vi "ExCenterStripSpecFwIN.vi"() -> ()   [LabVIEW 2010]
panel:
  in  "Filter":i16=1 min=1 max=100 step=1
  in  "Wavelength":dbl=546.0 format="%.2f"
  in  "Grating Speed":dbl=2000.0 min=1.0 step=1.0 format="%.2f"
  in  "Grating number":i16=1 min=1 max=100 step=1
  out "Strip":sgl[](graph)
  in  "Temperature":dbl=-10.0 format="%.2f"
  in  "Exposure":dbl=0.5 min=0.0 step=0.001 format="%.3f"
  in  "stop":bool
  out "error out":errorcluster
  in  "error in (no error)":errorcluster
  # "ExCenterStripSpecFwIN.vi (InSpectrum)\nCamera, Spectrometer and Filter Wheel control of the InSpectrum.  This vi will open the camera, spectrograph and filter wheel.  It will then move the grating to the Wavelength and set the filter.  Data will then be collected and displayed until the STOP button is hit."
  # "NOTES:\nA properly configured spectometer .ini must be present in the LabVIEW folder for spectrograph operation.\n\nConsult the Toolkit documentation for more information on how to configure this file."
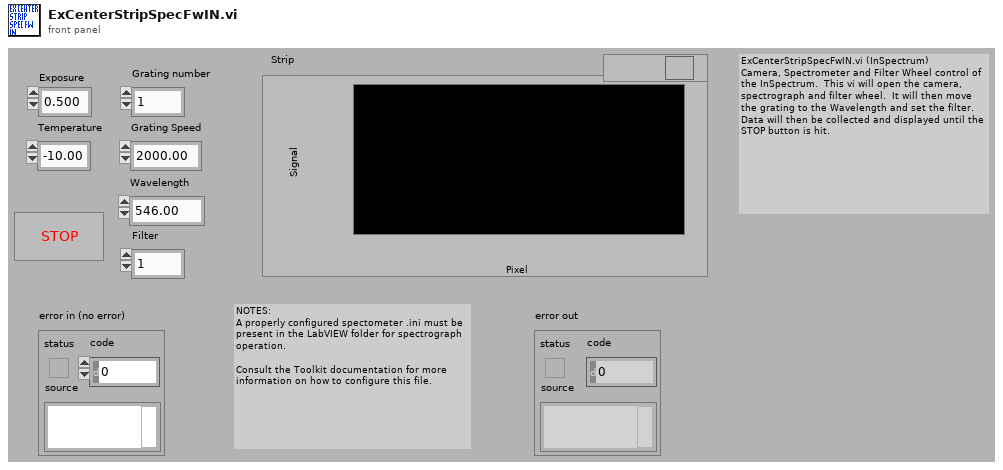
[diagram p1: front panel]
types:
  T1 = cluster{"acquire focus mode":u32, "Exposure":dbl, "Number of Images":u32, "Software accumulation":u32}
  T2 = cluster{"Camera Handle":u32, "Pulser Handle":u32, "File Handle":u32, "Display Handle":u32, "Image Handle":u32}
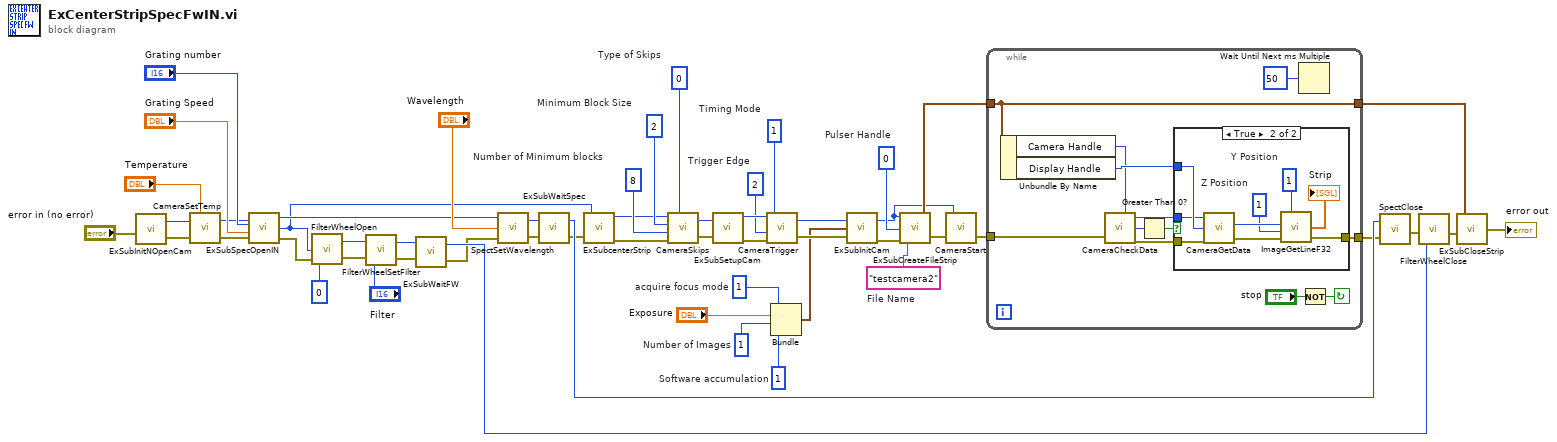
[diagram p0: block diagram]
diagram:
  w26 = u32 0  # Pulser Handle
  w31 = u32 1  # acquire focus mode
  w30 = u32 1  # Number of Images
  w29 = u32 1  # Software accumulation
  w28 = u32 1  # Timing Mode
  w32 = u32 2  # Trigger Edge
  w34 = u32 0  # Type of Skips
  w35 = u32 2  # Minimum Block Size
  w33 = u32 8  # Number of Minimum blocks
  w24 = "testcamera2"  # File Name
  n1 = call "ExSubInitNOpenCam.vi"("error in (no error)"="error in (no error)") -> ("Camera Handle"=w12:u32, "error out"=w13:errorcluster)
  n2 = call <userlib>:"CameraSetTemp.vi"("error in (no error)"=w13, "Temperature"="Temperature", "Camera Handle"=w12) -> ("error out"=w9:errorcluster, "Camera Handle"=w10:u32)
  n3 = call "ExSubSpecOpenIN.vi"("error in (no error)"=w9, "Grating speed"="Grating Speed", "Grating number"="Grating number", "Camera Handles"=w10) -> ("error out"=w18:errorcluster, "Camera Handle"=w16:u32, "Spectrometer Handle"=w38:u32)
  n4 = call <userlib>:"FilterWheelOpen.vi"("error in"=w18, "Device Handle"=w16, "Filter Wheel ID"=0) -> ("error out"=w17:errorcluster, "Filter Wheel Handlle"=w14:u32)
  n5 = call <userlib>:"FilterWheelSetFilter.vi"("error in"=w17, "Filter"="Filter", "Filter Wheel Handle"=w14) -> ("error out"=w7:errorcluster, "Filter Wheel Handle"=w5:u32)  [unwired: 1 in]
  n6 = call "ExSubWaitFW.vi"("error in (no error)"=w7, "Filter Wheel Handle"=w5) -> ("error out"=w6:errorcluster, "Filter Wheel handle"=w8:u32)
  n7 = call <userlib>:"SpectSetWavelength.vi"("error in"=w6, "Wavelength"="Wavelength", "Spectrometer Handle"=w38) -> ("error out"=w40:errorcluster, "Spectrumeter Handle"=w39:u32)
  n8 = call "ExSubWaitSpec.vi"("error in (no error)"=w40, "Spectrometer Handle"=w39) -> ("error out"=w23:errorcluster, "Spectrometer handle"=w37:u32)
  n9 = call "ExSubcenterStrip.vi"("error in (no error)"=w23, "Camera Handle"=w16) -> ("error out"=w21:errorcluster, "Camera Handle"=w22:u32)
  n10 = call <userlib>:"CameraSkips.vi"("Camera Handle"=w22, "Minimum Block Size"=w35, "Number of Minimum blocks"=w33, "error in"=w21, "Type of Skips"=w34) -> ("Camera Handle"=w46:u32, "error out"=w45:errorcluster)
  n11 = call "ExSubSetupCam.vi"("error in (no error)"=w45, "Camera Handle"=w46) -> ("error out"=w19:errorcluster, "Camera Handle"=w49:u32)
  n12 = call <userlib>:"CameraTrigger.vi"("error in"=w19, "Trigger Edge"=w32, "Timing Mode"=w28, "Camera Handle"=w49) -> ("error out"=w50:errorcluster, "Camera Handle"=w48:u32)
  n13 = Bundle("acquire focus mode"=w31, "Exposure"="Exposure", "Number of Images"=w30, "Software accumulation"=w29) -> (w27:T1)  [unwired: 1 in]
  n14 = call "ExSubInitCam.vi"("error in (no error)"=w50, "Camera Information"=w27, "Camera Handle"=w48) -> ("error out"=w20:errorcluster, "Camera Handle"=w25:u32)
  n15 = call "ExSubCreateFileStrip.vi"("error in (no error)"=w20, "File and Display Name"=w24, "Pulser Handle"=w26, "Camera Handle"=w25) -> ("error out"=w44:errorcluster, "Handles Out"=w52:T2)
  n16 = call <userlib>:"CameraStart.vi"("error in"=w44, "Camera Handle"=w25) -> ("error out"=w47:errorcluster)  [unwired: 1 out]
  n17 = while {
    tunnel: w52 -> [w63]
    tunnel: w47 -> [w62]
    tunnel: [w60] -> w36
    tunnel: [w63] -> w51
    stop <- w64 continue-if-true
    n18 = Unbundle By Name(w63) -> ("Camera Handle"=w55:u32, "Display Handle"=w59:u32)
    n19 = call <userlib>:"CameraCheckData.vi"("Camera Handle"=w55, "error in"=w62) -> ("Camera Handle"=w56:u32, "Number Of Frames Available"=w57:i32, "error out"=w61:errorcluster)
    n20 = Greater Than 0?(x=w57) -> (x > 0?=w58:bool)
    n21 = case shown="True" w58 {
      tunnel: w61 -> [w67 w75]
      tunnel: [w67 w73] -> w60
      tunnel: w59 -> [_ w71]
      tunnel: w56 -> [_ w70]
      frame False {
      }
      frame True {
        w68 = u32 1  # Z Position
        w69 = u32 1  # Y Position
        n22 = call <userlib>:"CameraGetData.vi"("error in"=w75, "Data Handle"=w71, "Camera Handle"=w70) -> ("error out"=w74:errorcluster, "Data Handle"=w72:u32)  [unwired: 1 out]
        n23 = call <userlib>:"ImageGetLineF32.vi"("error in"=w74, "Z Position"=w68, "Y Position"=w69, "Data Handle"=w72) -> ("error out"=w73:errorcluster, "Array F32"=→"Strip":sgl[])  [unwired: 1 out]
      }
    }
    n24 = Wait Until Next ms Multiple(millisecond multiple=u32 50) -> ()  [unwired: 1 out]
    n25 = Not(x="stop") -> (.not. x?=w64:bool)
  }
  n26 = call <userlib>:"SpectClose.vi"("error in"=w36, "Spectrometer Handle"=w37) -> ("error out"=w3:errorcluster)
  n27 = call <userlib>:"FilterWheelClose.vi"("error in"=w3, "Filter Wheel Handle"=w8) -> ("error out"=w2:errorcluster)
  n28 = call "ExSubCloseStrip.vi"("error in (no error)"=w2, "Handles In"=w51) -> ("error out"=→"error out":errorcluster)
